vi "New Logger_1.vi"(4 "dialog on failure? (T)":bool=TRUE, 5 "minimum log level (Info)":T1=enum."Info", 6 "enabled? (T)":bool=TRUE, 8 "error in (no error)":errorcluster, 9 "log handler (file handler)":refnum<class "Formatting Handler.lvclass">, 10 "log filter (none)":refnum<class "Filter.lvclass">, 11 "logger scope (all)":refnum<class "Scope.lvclass">) -> (0 "error out":errorcluster, 3 "logger":refnum<class "Logger.lvclass">)   [LabVIEW 2018]
uses:
  src/api/logger_class/Logger.lvclass
  src/api/configuration/handlers/file_handler/File Handler.lvclass
  src/api/extension/formatting_handler_interface/Formatting Handler.lvclass
  src/api/extension/scope_interface/Scope.lvclass
  src/api/extension/filter_interface/Filter.lvclass
  src/api/logger_class/Log Levels.ctl
panel:
  # "Connector Pane"
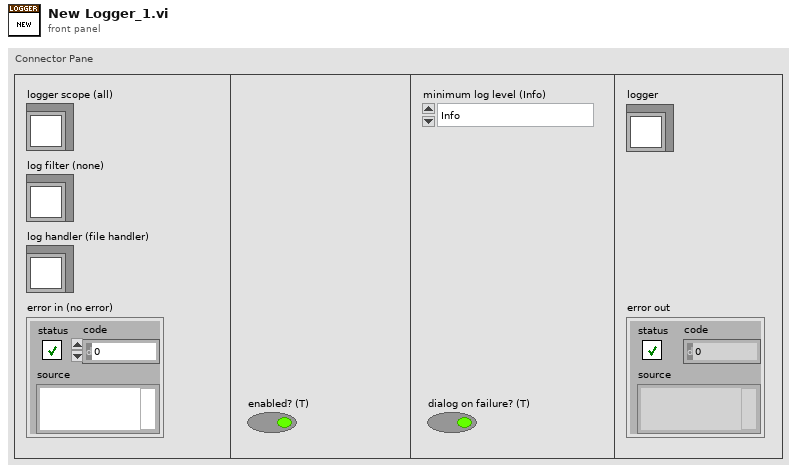
[diagram p1: front panel]
types:
  T1 = typedef "GLog.lvlib/Logger.lvclass/Log Levels.ctl" = enum16{"Trace", "Debug", "Info", "Warning", "Error", "Critical"}
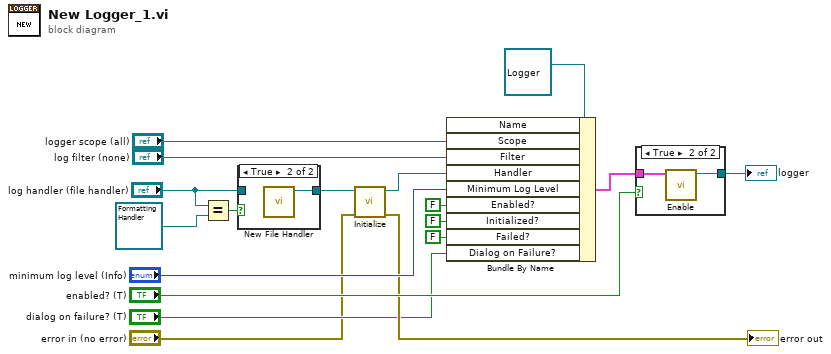
[diagram p0: block diagram]
diagram:
  n1 = Equal?(x="log handler (file handler)", y=refnum<class "Formatting Handler.lvclass"> refnum ("log handler (file handler)")) -> (x = y?=w1:bool)
  n2 = case shown="True" w1 {
    tunnel: [w19 w20] -> w14
    tunnel: "log handler (file handler)" -> [w19 _]
    frame False {
    }
    frame True {
      n3 = call "New File Handler.vi"() -> ("file handler"=w20:refnum<class "File Handler.lvclass">)  [unwired: 11 in]
    }
  }
  n4 = call-dynamic "Initialize.vi"("error in (no error)"="error in (no error)", "handler in"=w14) -> ("error out"=→"error out":errorcluster, "handler out"=w12:refnum<class "Formatting Handler.lvclass">)  [unwired: 8 in]
  n5 = Bundle By Name(cluster=refnum<class "Logger.lvclass"> refnum ("logger"), "Scope"="logger scope (all)", "Filter"="log filter (none)", "Handler"=w12, "Minimum Log Level"="minimum log level (Info)", "Enabled?"=FALSE ("Active?"), "Initialized?"=FALSE ("Active?"), "Failed?"=FALSE, "Dialog on Failure?"="dialog on failure? (T)") -> (w8:cluster{})  [unwired: 1 in]
  n6 = case shown="True" "enabled? (T)" {
    tunnel: w8 -> [w21 w23]
    tunnel: [w21 w22] -> w7
    frame False {
    }
    frame True {
      n7 = call "Enable.vi"("logger in"=w23) -> ("logger out"=w22:refnum<class "Logger.lvclass">)  [unwired: 10 in]
    }
  }
  "logger" <- w7
